vi "FunctDataMgr.Update SN.vi"(8 "error in (no error)":errorcluster, 10 "SN":string, 11 "FunctDataMgr in":refnum<class "FunctDataMgr.lvclass">) -> (0 "error out":errorcluster, 3 "FunctDataMgr out":refnum<class "FunctDataMgr.lvclass">)   [LabVIEW 2018, in "FunctDataMgr.lvclass"]
uses:
  FunctDataMgr.lvclass
  FunctDataMgr.lvclass/FunctDataMgr.ctl
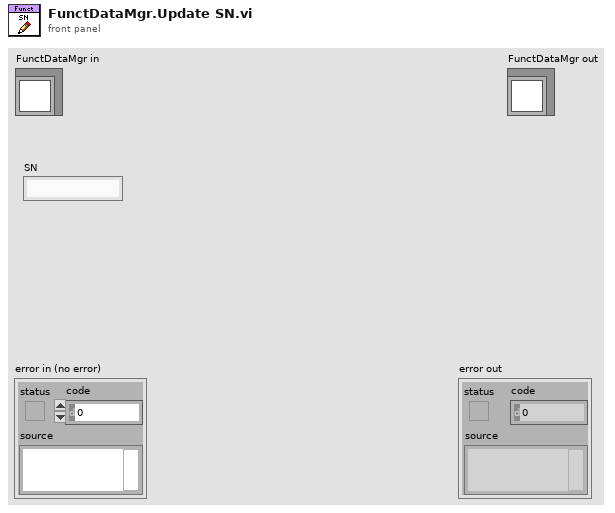
[diagram p1: front panel]
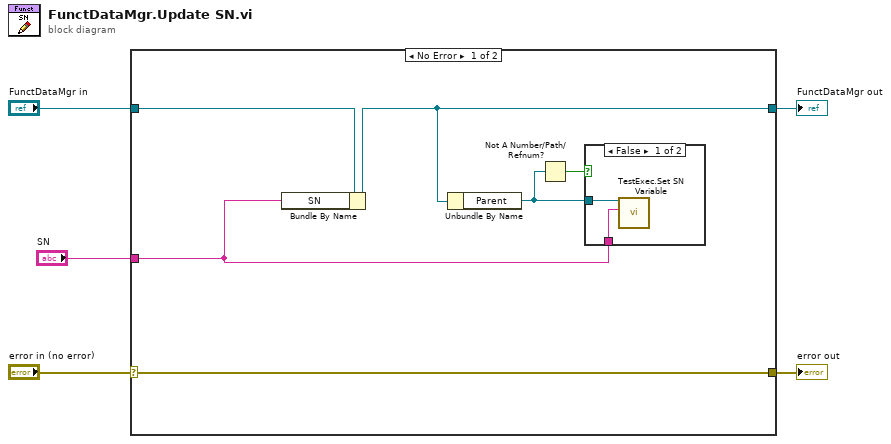
[diagram p0: block diagram]
diagram:
  n1 = case shown="No Error" "error in (no error)" {
    selector: "error in (no error)" -> [w11 w15]
    tunnel: [w11 w15] -> w4
    tunnel: [w9 w14] -> w2
    tunnel: "FunctDataMgr in" -> [w10 w14]
    tunnel: "SN" -> [w7 _]
    frame No Error {
      n2 = Bundle By Name(cluster=w10, "SN"=w7) -> (w9:refnum<class "FunctDataMgr.lvclass">)
      n3 = Unbundle By Name(w9) -> ("Parent"=w8:refnum<queue>)
      n4 = Not A Number/Path/Refnum?(number/path/refnum=w8) -> (NaN/Path/Refnum?=w6:bool)
      n5 = case shown="False" w6 {
        tunnel: w8 -> [w13 _]
        tunnel: w7 -> [w12 _]
        frame False {
          n6 = call "TestExec.Set SN Variable.vi"("Sn"=w12, "Q In"=w13) -> ()  [unwired: 8 in, 2 out]
        }
        frame True {
        }
      }
    }
    frame Error {
    }
  }
  "error out" <- w4
  "FunctDataMgr out" <- w2
